vi "03 - Calling MATLAB.vi"() -> ()   [LabVIEW 2026]
panel:
  out "Fractal Plot":dbl[][](graph)
  in  "m [kg]":dbl=9.11e-31
  in  "L [nm]":dbl(slide)=2.0 scale=1e-06..2.0
  in  "V0 [eV]":dbl(slide)=10.000000000000002 scale=10.0..10000.0
  in  "Quantum Number":i32(slide)=1 scale=1.0..100.0
  out "Wave Function":cluster{"x":dbl[], "y":dbl[]}(graph)
  out "Probability Density":cluster{"x":dbl[], "y":dbl[]}(graph)
  out "E [eV]":dbl
  in  "Stop":bool
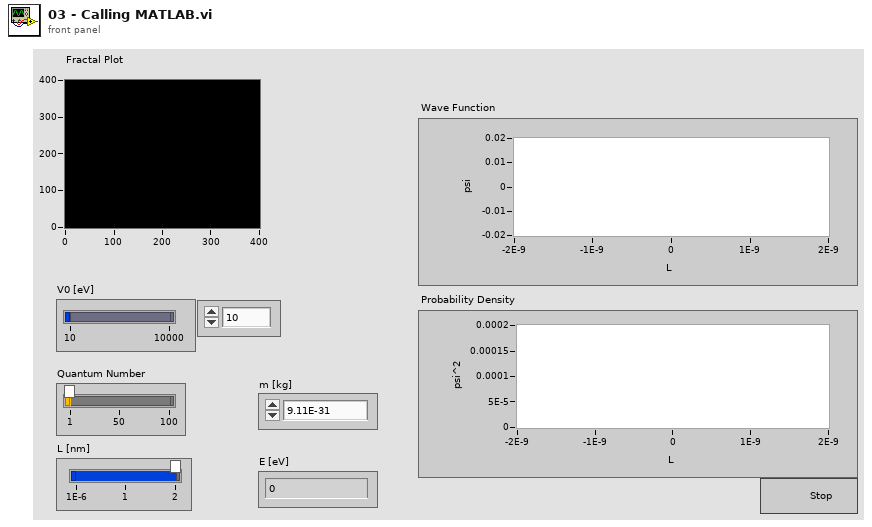
[diagram p1: front panel]
types:
  T1 = cluster{"E [eV]":dbl, "Wave Function":cluster{"x":dbl[], "y":dbl[]}, "Probability Density":cluster{"x":dbl[], "y":dbl[]}}
  T2 = cluster{"R":dbl, "L":dbl, "hbar":dbl, "V0":dbl, "m":dbl}
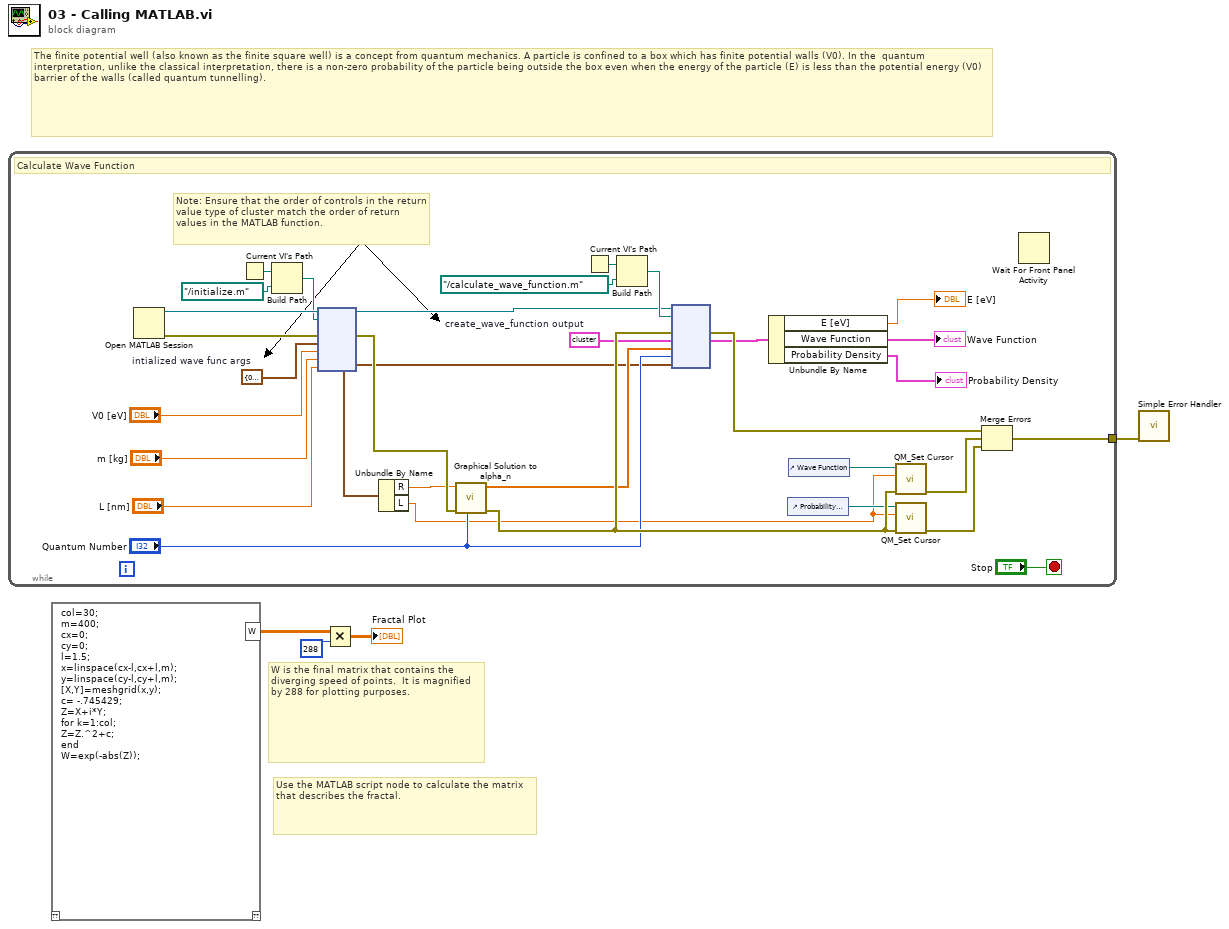
[diagram p0: block diagram]
diagram:
  # "The finite potential well (also known as the finite square well) is a concept from quantum mechanics. A particle is confined to a box which has finite potential walls (V0). In the  quantum interpretation, unlike the classical interpretation, there is a non-zero probability of the particle being outside the box even when the energy of the particle (E) is less than the potential energy (V0) barrier of the walls (called quantum tunnelling)."
  # "Use the MATLAB script node to calculate the matrix that describes the fractal."
  # "W is the final matrix that contains the diverging speed of points.  It is magnified by 288 for plotting purposes."
  n1 = while {
    tunnel: [w34] -> w4
    stop <- "Stop" stop-if-true
    w15 = T1 {"E [eV]"=0.0, "Wave Function"={"x"=array[30003 elements], "y"=array[30003 elements]}, "Probability Density"={"x"=array[30003 elements], "y"=array[30003 elements]}}  # create_wave_function output
    w6 = T2 {"R"=0.0, "L"=0.0, "hbar"=0.0, "V0"=0.0, "m"=0.0}  # intialized wave func args
    # "Note: Ensure that the order of controls in the return value type of cluster match the order of return values in the MATLAB function."
    # "Calculate Wave Function"
    n2 = Open MATLAB Session() -> (8:w26:refnum<k37>, 11:w33:errorcluster)  [unwired: 2 in]
    n3 = Current VI's Path() -> (path=w25:path)
    n4 = Build Path(base path=w25, name or relative path=path "../initialize.m") -> (appended path=w23:path)
    n5 = node(w26, w23, w33, w6, "V0 [eV]", "m [kg]", "L [nm]") -> (w16:refnum<k37>, w32:errorcluster, w5:T2)  [unwired: 4 in, 2 out]
    n6 = Unbundle By Name(w5) -> ("R"=w11:dbl, "L"=w10:dbl)
    n7 = call "Graphical Solution to alpha_n.vi"("Quantum Number"="Quantum Number", "error in"=w32, "R"=w11) -> ("error out"=w30:errorcluster, "alpha_n"=w14:dbl[])  [unwired: 6 in, 1 out]
    n8 = Current VI's Path() -> (path=w18:path)
    n9 = Build Path(base path=w18, name or relative path=path "../calculate_wave_function.m") -> (appended path=w17:path)
    n10 = node(w16, w17, w30, w15, w14, "Quantum Number", w5) -> (w31:errorcluster, w13:T1)  [unwired: 4 in, 3 out]
    n11 = Unbundle By Name(w13) -> ("E [eV]"=→"E [eV]":dbl, "Wave Function"=→"Wave Function":cluster{"x":dbl[], "y":dbl[]}, "Probability Density"=→"Probability Density":cluster{"x":dbl[], "y":dbl[]})
    n12 = control-ref of="Probability Density"() -> (w28:refnum<vi>)
    n13 = control-ref of="Wave Function"() -> (w29:refnum<vi>)
    n14 = call "QM_Set Cursor.vi"("error in (no error)"=w30, "L"=w10, "XYGraph in"=w29) -> ("error out"=w36:errorcluster)  [unwired: 8 in]
    n15 = call "QM_Set Cursor.vi"("error in (no error)"=w30, "L"=w10, "XYGraph in"=w28) -> ("error out"=w35:errorcluster)  [unwired: 8 in]
    n16 = Merge Errors(w31, w36, w35) -> (w34:errorcluster)
    n17 = Wait For Front Panel Activity() -> ()  [unwired: 3 in, 1 out]
  }
  n18 = script code="col=30;\nm=400;\ncx=0;\ncy=0;\nl=1.5;\nx=linspace(cx-l,cx+l,m);\ny=linspace(cy-l,cy+l,m);\n[X,Y]=meshgrid(x,y);\nc= -.745429;\nZ=X+i*Y;\nfor k=1:col;\nZ=Z.^2+c;\nend\nW=exp(-abs(Z));"() -> ("W"=w1:dbl[][])  [unwired: 1 in, 1 out]
  n19 = Multiply(x=w1, y=288) -> (x*y=→"Fractal Plot":dbl[][])
  n20 = call <vilib>:"Simple Error Handler.vi"("error in (no error)"=w4) -> ()  [unwired: 4 in, 5 out]
